vi "Get SubVI References.vi"(8 "error in (no error)":errorcluster, 11 "Owner vi in":refnum<vi>) -> (0 "error out":errorcluster, 2 "SubVI refs":refnum<vi>[](array[refnum]), 3 "Owner vi out":refnum<vi>)   [LabVIEW 2019, in "gRPC Template Creation Utility.lvlib"]
uses:
  gRPC Template Creation Utility.lvlib
  <vilib>/Utility/traverseref.llb/TRef TravTarget.ctl
  <vilib>/Utility/traverseref.llb/VI Scripting - Traverse.lvlib
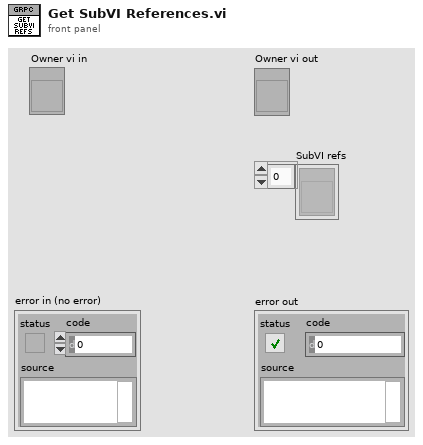
[diagram p1: front panel]
types:
  T1 = typedef "TRef TravTarget.ctl" = enum16{"FP", "BD", "Other"}
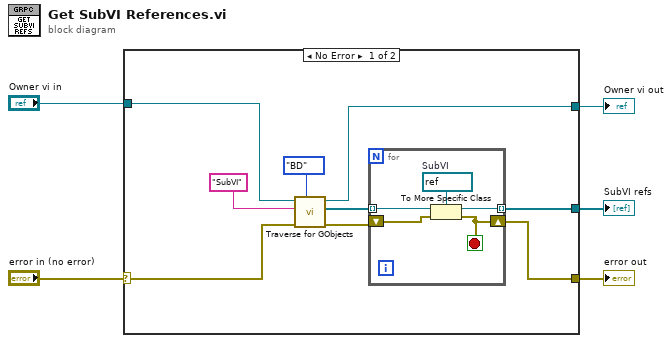
[diagram p0: block diagram]
diagram:
  n1 = case shown="No Error" "error in (no error)" {
    selector: "error in (no error)" -> [w7 w21]
    tunnel: [w14 _] -> w5
    tunnel: "Owner vi in" -> [w11 w20]
    tunnel: [w8 w20] -> w3
    tunnel: [w6 w21] -> w1
    frame No Error {
      n2 = call <vilib>:"Traverse for GObjects.vi"("Traverse Target"=TRef_TravTarget."BD", "error in (no error)"=w7, "Class Name"="SubVI", "VI Refnum"=w11) -> ("error out"=w13:errorcluster, "References"=w12:refnum<vi>[], "dup VI Refnum"=w8:refnum<vi>)  [unwired: 4 in, 1 out]
      n3 = for {
        tunnel: w12 -> [w18] mode=indexing
        tunnel: [w16] -> w14 mode=indexing
        shift-right: [w15] -> w6
        shift-left: w13 -> [w17]
        stop <- w15 stop-if-true
        w19 = refnum<vi> refnum  # SubVI
        n4 = To More Specific Class(target class=w19, reference=w18, error in=w17) -> (specific class reference=w16:refnum<vi>, error out=w15:errorcluster)
      }
    }
    frame Error {
    }
  }
  "SubVI refs" <- w5
  "Owner vi out" <- w3
  "error out" <- w1
